vi "splitFractionalSeconds[ms].vi"(10 "(Integer) Time (ms)":i64, 11 "Epoch in":refnum<class "Epoch.lvclass">) -> (1 "Fractional Second":dbl format="%#.6f", 2 "(Integer) Time (s)":i64, 3 "Epoch out":refnum<class "Epoch.lvclass">)   [LabVIEW 2013, in "Epoch.lvclass"]
uses:
  Epoch.lvclass
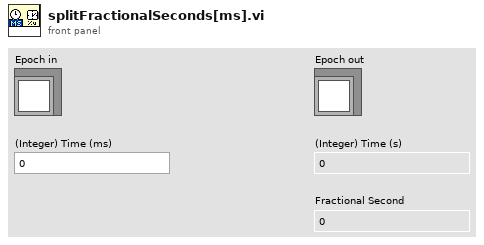
[diagram p1: front panel]
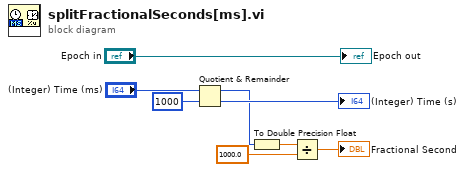
[diagram p0: block diagram]
diagram:
  n1 = Quotient & Remainder(x="(Integer) Time (ms)", y=i64 1000) -> (x-y*floor(x/y)=w4:i64, floor(x/y)=→"(Integer) Time (s)":i64)
  n2 = To Double Precision Float(number=w4) -> (double precision float=w2:dbl)
  n3 = Divide(x=w2, y=1000.0) -> (x/y=→"Fractional Second":dbl)
  "Epoch out" <- "Epoch in"
